vi "Write_currentNumber.vi"(8 "error in (no error)":errorcluster, 10 "currentNumber":i32, 11 "FactoryTcpServer in":refnum<class "FactoryTcpServer.lvclass">) -> (0 "error out":errorcluster, 3 "FactoryTcpServer out":refnum<class "FactoryTcpServer.lvclass">)   [LabVIEW 2018, in "FactoryTcpServer.lvclass"]
doc: "Write the currentNumber."
uses:
  FactoryTcpServer.lvclass
  FactoryTcpServer.lvclass/FactoryTcpServer.ctl
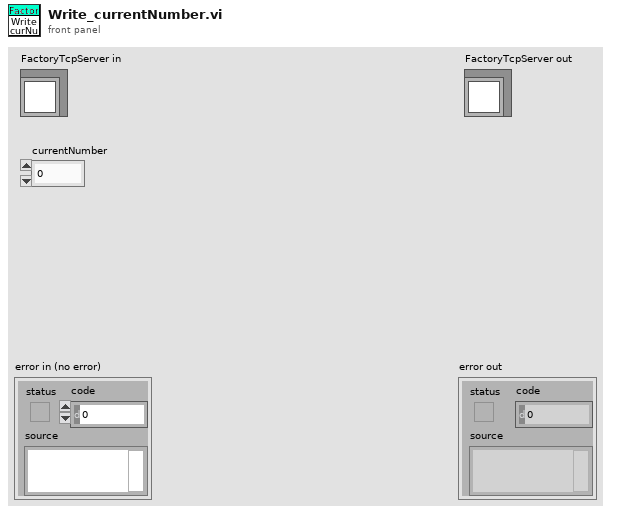
[diagram p1: front panel]
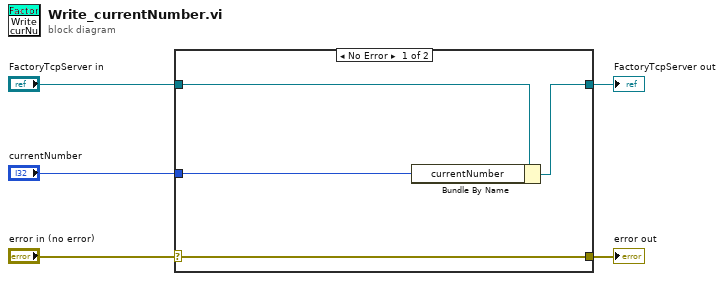
[diagram p0: block diagram]
diagram:
  n1 = case shown="No Error" "error in (no error)" {
    selector: "error in (no error)" -> [w9 w10]
    tunnel: [w9 w10] -> w4
    tunnel: [w7 w11] -> w2
    tunnel: "FactoryTcpServer in" -> [w8 w11]
    tunnel: "currentNumber" -> [w6 _]
    frame No Error {
      n2 = Bundle By Name(cluster=w8, "currentNumber"=w6) -> (w7:refnum<class "FactoryTcpServer.lvclass">)
    }
    frame Error {
    }
  }
  "error out" <- w4
  "FactoryTcpServer out" <- w2
